vi "get index type definitions.vi"(11 "fixed channel configuration in":refnum<class "fixed channel configuration.lvclass">) -> (2 "index type defs":T1, 3 "fixed channel configuration out":refnum<class "fixed channel configuration.lvclass">)   [LabVIEW 2013, in "fixed channel configuration.lvclass"]
uses:
  fixed channel configuration.lvclass
  index type definitions.ctl
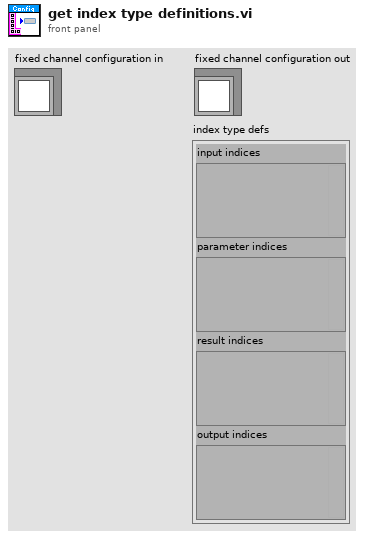
[diagram p1: front panel]
types:
  T1 = typedef "fixed channel configuration.lvclass/index type definitions.ctl" = cluster{"input indices":variant, "parameter indices":variant, "result indices":variant, "output indices":variant}
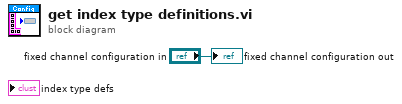
[diagram p0: block diagram]
diagram:
  "fixed channel configuration out" <- "fixed channel configuration in"
